vi "Automated Kitty Litter Box VI.vi"() -> ()   [LabVIEW 2021]
uses:
  <vilib>/LabVIEW Hacker/LINX/Private/Device/Type Defs/Stimulus Pulse.ctl
  <vilib>/LabVIEW Hacker/LINX/Public/Peripherals/Digital/Digital Write 1 Chan.vi
  <vilib>/Quanser/Rapid Control Prototyping Toolkit/hardware/HIL Board/_TypeSpecific/HIL Read Analog (Scalar).vi
  <vilib>/LabVIEW Hacker/LINX/LVH-LINX.lvlib
  <vilib>/Quanser/Rapid Control Prototyping Toolkit/hardware/HIL Board/HIL Board.lvclass
  <vilib>/LabVIEW Hacker/LINX/Private/Device/Device.lvlib
panel:
  out "Waveform Chart":dbl(graph)
  out "Rev":dbl
  out "Count":i32
  in  "stop":bool
  out "Distance (inches)":u32 format="%.2f"
  in  "Serial Port":refnum<visa-resource-name>="N/A"
  out "Saved Value":dbl
  out "Force Sensor Output":dbl
  # "FORCE SENSOR"
  # "MAIN MOTOR HALL EFFECT SENSOR"
  # "ULTRASONIC SENSOR"
  # "ARDUINO INITIALIZATION"
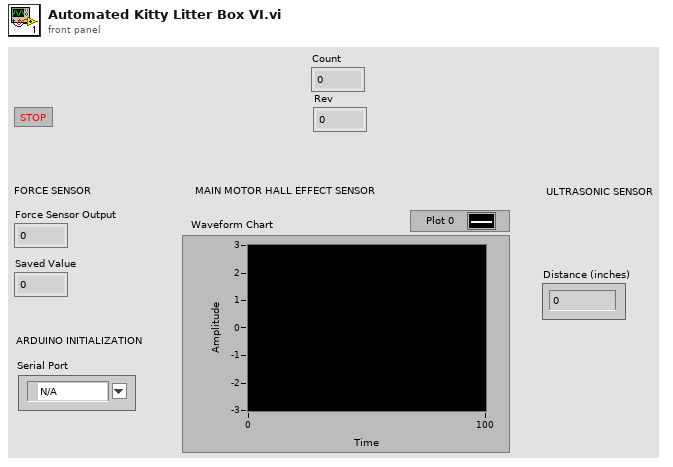
[diagram p1: front panel]
types:
  T1 = typedef "LVH-LINX.lvlib/LINX Ref.ctl" = cluster{"Platform":T2, "Interface":T3, "LINX Device Config":T4}
  T2 = typedef "LVH-LINX.lvlib/Platform.ctl" = enum16{"LINX", "myRIO"}
  T3 = typedef "LVH-LINX.lvlib/Interface.ctl" = enum16{"Serial", "TCP"}
  T4 = typedef "LVH-LINX.lvlib/Device.lvlib/LINX Device Config.ctl" = cluster{"Interface":T3, "COM Port":refnum<visa-resource-name>, "TCP Configuration":T5, "Device Family":T6, "Device ID":u8, "Device Name":string, "TCP Ref":refnum<k5>}
  T5 = typedef "LVH-LINX.lvlib/Device.lvlib/TCP Config.ctl" = cluster{"IP Address":string, "Port":u16}
  T6 = typedef "LVH-LINX.lvlib/Device Family.ctl" = enum8{"National Instruments", "Digilent", "Arduino"}
  T7 = typedef "LVH-LINX.lvlib/Device.lvlib/Stimulus Pulse.ctl" = enum16{"None", "Active Low", "Active High"}
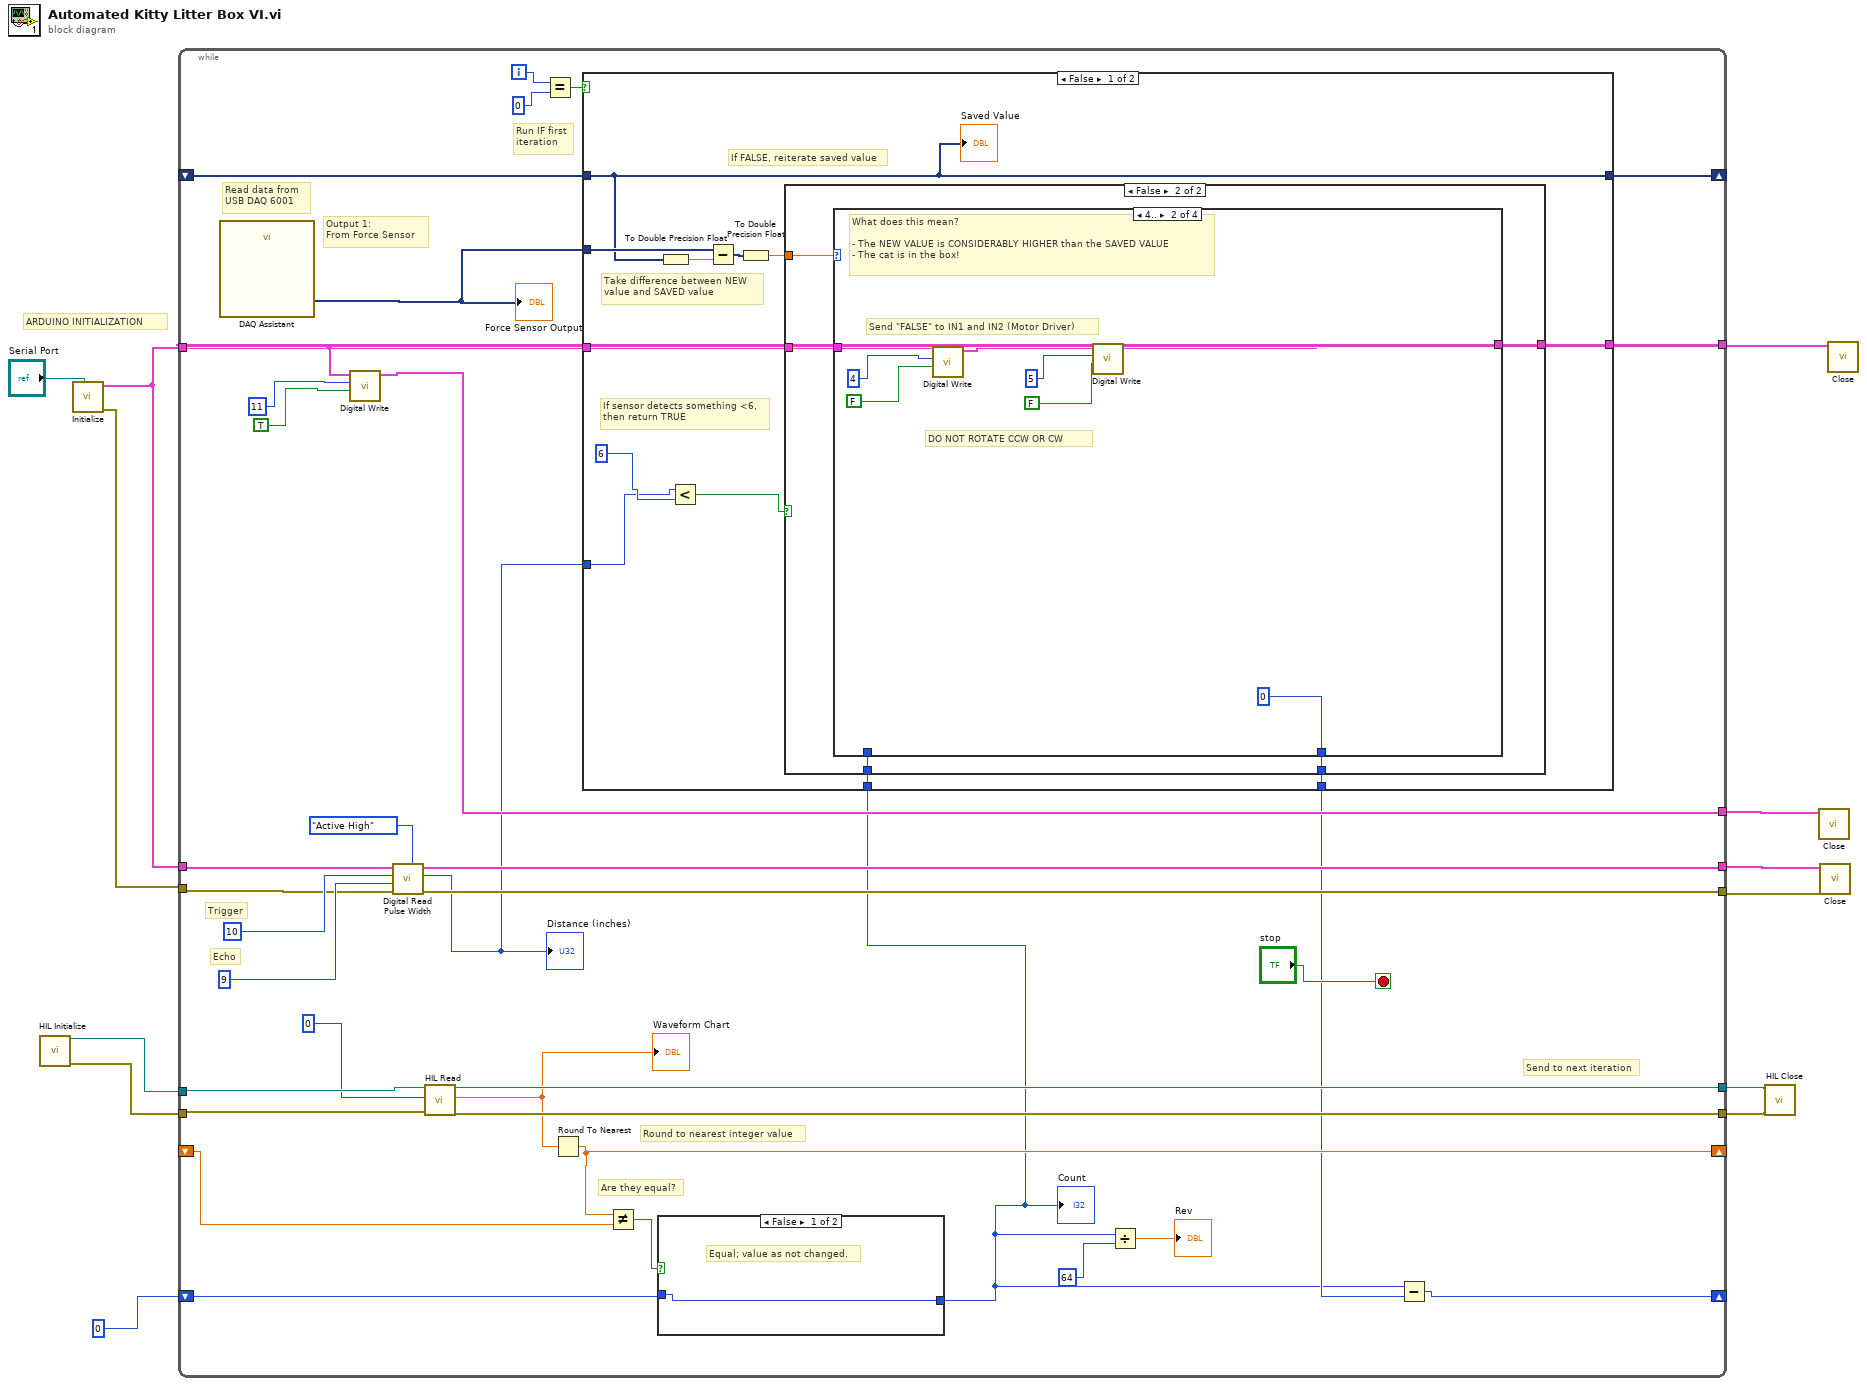
[diagram p0: block diagram]
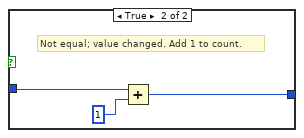
[diagram p2: hidden frame]
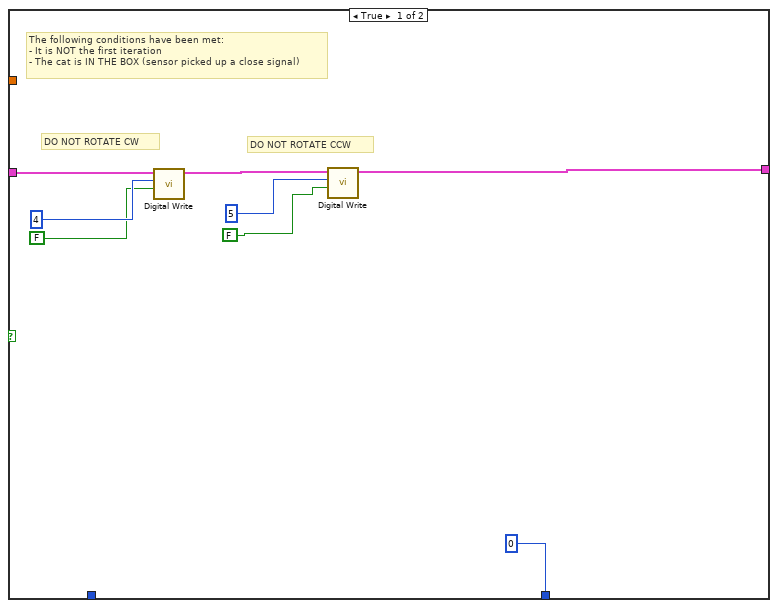
[diagram p3: hidden frame]
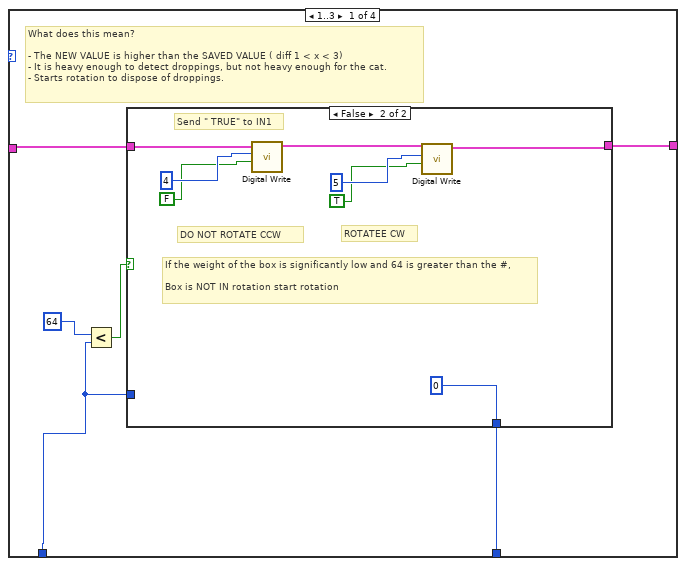
[diagram p4: hidden frame]
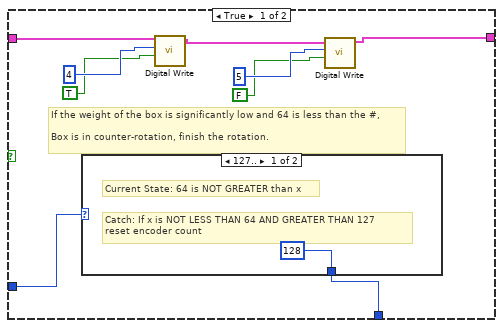
[diagram p5: hidden frame]
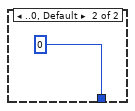
[diagram p6: hidden frame]
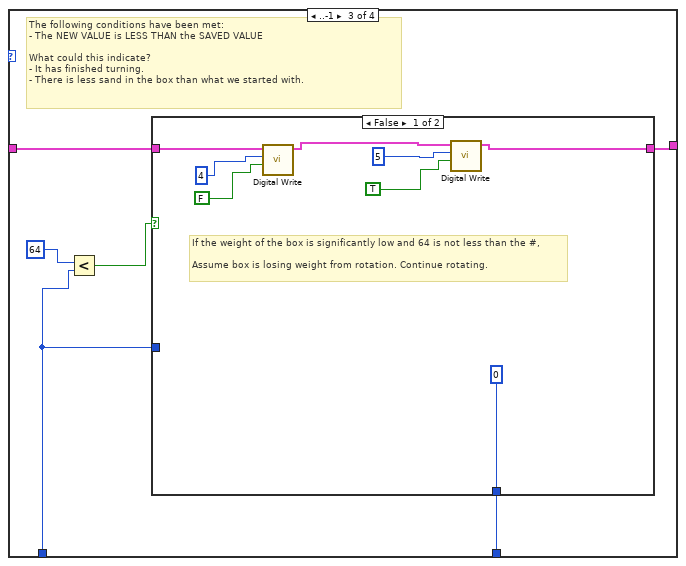
[diagram p7: hidden frame]
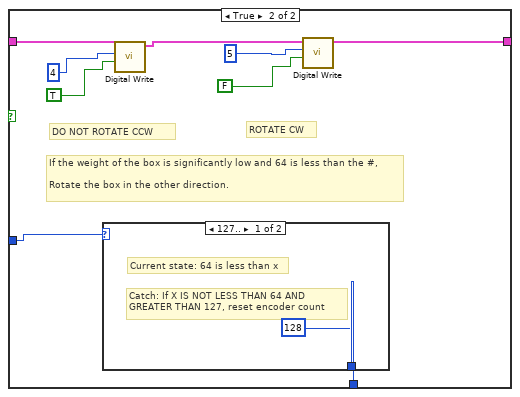
[diagram p8: hidden frame]
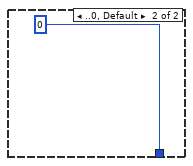
[diagram p9: hidden frame]
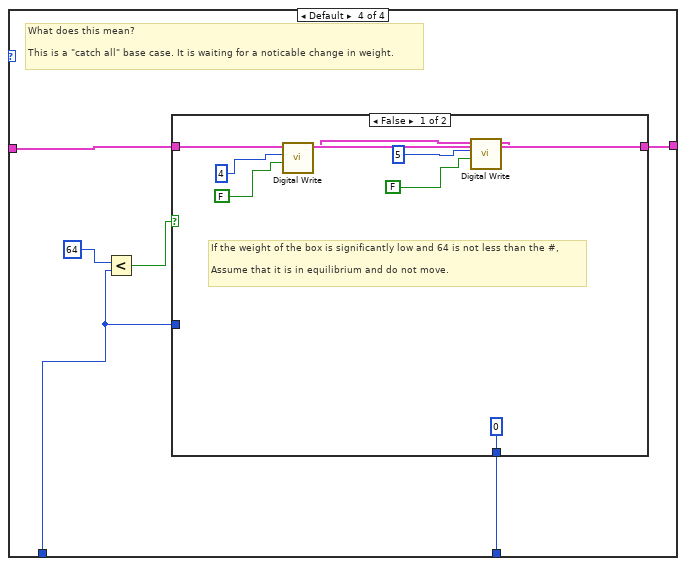
[diagram p10: hidden frame]
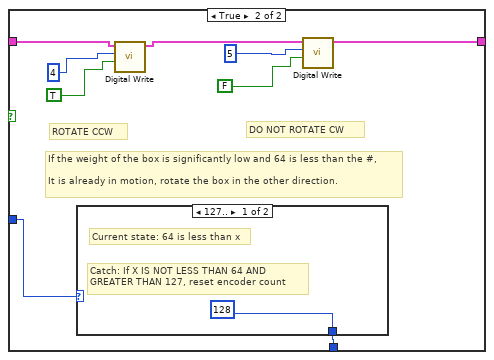
[diagram p11: hidden frame]
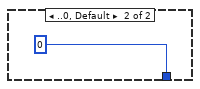
[diagram p12: hidden frame]
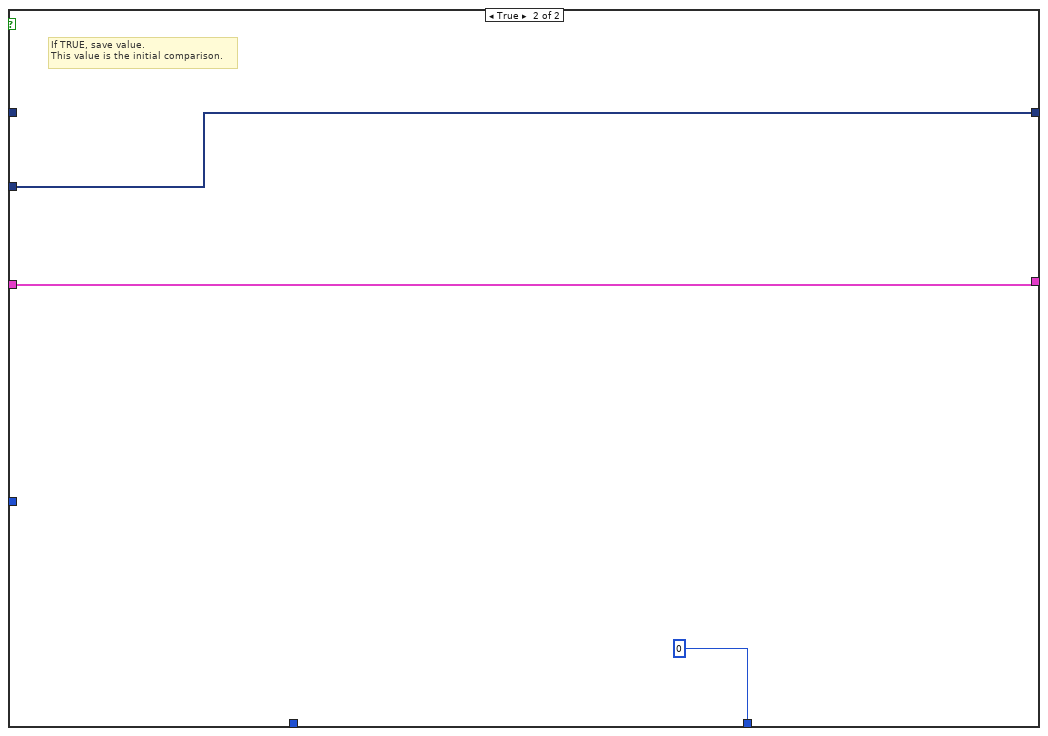
[diagram p13: hidden frame]
diagram:
  # "ARDUINO INITIALIZATION"
  n1 = call "HIL Initialize"() -> ("board out"=w5:refnum<class "HIL Board.lvclass">, "error out"=w4:errorcluster)  [unwired: 14 in]
  n2 = call <vilib>:"Initialize.vi"("Serial Port"="Serial Port") -> ("Error Out"=w8:errorcluster, "LINX Ref"=w10:T1)  [unwired: 8 in, 1 out]
  n3 = while {
    shift-right: [w44] -> _
    shift-left: _ -> [w43]
    tunnel: w10 -> [w27]
    tunnel: [w26] -> w7
    shift-right: [w15] -> _
    shift-left: 0 -> [w41]
    tunnel: w10 -> [w35]
    tunnel: [w34] -> w9
    tunnel: w8 -> [w23]
    tunnel: [w33] -> w6
    tunnel: w5 -> [w32]
    tunnel: w4 -> [w30]
    tunnel: [w29] -> w2
    tunnel: [w28] -> w3
    tunnel: [w22] -> w1
    shift-right: [w18] -> _
    shift-left: _ -> [w17]
    i -> [w47]
    stop <- "stop" stop-if-true
    # "Are they equal?"
    # "Send to next iteration"
    # "Round to nearest integer value"
    # "Trigger"
    # "Echo"
    # "Run IF first\niteration"
    # "Output 1:\nFrom Force Sensor"
    # "Read data from \nUSB DAQ 6001"
    n4 = call "DAQ Assistant"() -> ("data"=w38:dynamicdata)  [unwired: 17 in, 2 out]
    "Force Sensor Output" <- w38
    n5 = call-poly <vilib>:"Digital Write.vi"("Output Value"=TRUE, "DO Channel"=u8 11, "LINX Resource"=w35) -> ("LINX Resource"=w34:T1)  [unwired: 7 in, 1 out]
    n6 = call <vilib>:"Digital Read Pulse Width.vi"("Stimulus Pulse (Active High)"=Stimulus_Pulse."Active High", "Error In"=w23, "DO Channel"=9, "DI Channel"=10, "LINX Resource"=w27) -> ("Error Out"=w22:errorcluster, "Pulse Width (uS)"=w20:u32, "LINX Resource"=w26:T1)  [unwired: 4 in]
    "Distance (inches)" <- w20
    n7 = call-poly <vilib>:"HIL Read.vi"("board in"=w32, "channel"=0, "error in (no error)"=w30) -> ("board out"=w28:refnum<class "HIL Board.lvclass">, "voltage"=w19:dbl, "error out"=w29:errorcluster)  [unwired: 14 in]
    "Waveform Chart" <- w19
    n8 = Equal?(x=w47, y=0) -> (x = y?=w45:bool)
    n9 = Round To Nearest(number=w19) -> (nearest integer value=w18:dbl)
    n10 = Not Equal?(x=w18, y=w17) -> (x != y?=w16:bool)
    n11 = case shown="False" w16 {
      tunnel: [w48 w50] -> w13
      tunnel: w41 -> [w48 w49]
      frame False {
        # "Equal; value as not changed."
      }
      frame True {
        # "Not equal; value changed. Add 1 to count."
        n12 = Add(x=w49, y=1) -> (x+y=w50:i32)
      }
    }
    "Count" <- w13
    n13 = case shown="False" w45 {
      tunnel: w38 -> [w63 w161]
      tunnel: [w61 w161] -> w44
      tunnel: w43 -> [w61 _]
      tunnel: w35 -> [w58 w160]
      tunnel: w20 -> [w55 _]
      tunnel: [w54 w160] -> w33
      tunnel: w13 -> [w53 _]
      tunnel: [w52 0] -> w14
      frame False {
        # "If sensor detects something <6,\nthen return TRUE"
        # "Take difference between NEW\nvalue and SAVED value"
        # "If FALSE, reiterate saved value"
        n14 = To Double Precision Float(number=w61) -> (double precision float=w62:dbl)
        n15 = Less?(x=w55, y=6) -> (x < y?=w57:bool)
        n16 = Subtract(x=w63, y=w62) -> (x-y=w60:dynamicdata)
        n17 = To Double Precision Float(number=w60) -> (double precision float=w59:dbl)
        n18 = case shown="False" w57 {
          tunnel: w59 -> [_ w76]
          tunnel: w58 -> [w68 w75]
          tunnel: [w66 w74] -> w54
          tunnel: w53 -> [_ w73]
          tunnel: [0 w72] -> w52
          frame True {
            # "The following conditions have been met:\n- It is NOT the first iteration\n- The cat is IN THE BOX (sensor picked up a close signal)"
            # "DO NOT ROTATE CCW"
            # "DO NOT ROTATE CW"
            n19 = call-poly <vilib>:"Digital Write.vi"("Output Value"=FALSE, "DO Channel"=u8 4, "LINX Resource"=w68) -> ("LINX Resource"=w67:T1)  [unwired: 7 in, 1 out]
            n20 = call-poly <vilib>:"Digital Write.vi"("Output Value"=FALSE, "DO Channel"=u8 5, "LINX Resource"=w67) -> ("LINX Resource"=w66:T1)  [unwired: 7 in, 1 out]
          }
          frame False {
            n21 = case shown="4.." w76 {
              tunnel: w75 -> [w82 w108 w115 w137]
              tunnel: [w81 w109 w114 w137] -> w74
              tunnel: w73 -> [w77 _ w110 w135]
              tunnel: [w78 0 w111 w136] -> w72
              frame 1..3 {
                # "What does this mean?\n\n- The NEW VALUE is higher than the SAVED VALUE ( diff 1 < x < 3)\n- It is heavy enough to detect droppings, but not heavy enough for the cat.\n- Starts rotation to dispose of droppings."
                n22 = Less?(x=64, y=w77) -> (x < y?=w79:bool)
                n23 = case shown="False" w79 {
                  tunnel: w82 -> [w87 w101]
                  tunnel: [w85 w95] -> w81
                  tunnel: [w84 0] -> w78
                  tunnel: w77 -> [w83 _]
                  frame True {
                    # "If the weight of the box is significantly low and 64 is less than the #,\n\nBox is in counter-rotation, finish the rotation."
                    n24 = case shown="127.." w83 {
                      tunnel: [128 0] -> w84
                      frame 127.. {
                        # "Current State: 64 is NOT GREATER than x"
                        # "Catch: If x is NOT LESS THAN 64 AND GREATER THAN 127\nreset encoder count"
                      }
                      frame ..0, Default {
                      }
                    }
                    n25 = call-poly <vilib>:"Digital Write.vi"("Output Value"=TRUE, "DO Channel"=u8 4, "LINX Resource"=w87) -> ("LINX Resource"=w86:T1)  [unwired: 7 in, 1 out]
                    n26 = call-poly <vilib>:"Digital Write.vi"("Output Value"=FALSE, "DO Channel"=u8 5, "LINX Resource"=w86) -> ("LINX Resource"=w85:T1)  [unwired: 7 in, 1 out]
                  }
                  frame False {
                    # "If the weight of the box is significantly low and 64 is greater than the #,\n\nBox is NOT IN rotation start rotation"
                    # "ROTATEE CW"
                    # "DO NOT ROTATE CCW"
                    # "Send \" TRUE\" to IN1"
                    n27 = call-poly <vilib>:"Digital Write.vi"("Output Value"=FALSE, "DO Channel"=u8 4, "LINX Resource"=w101) -> ("LINX Resource"=w96:T1)  [unwired: 7 in, 1 out]
                    n28 = call-poly <vilib>:"Digital Write.vi"("Output Value"=TRUE, "DO Channel"=u8 5, "LINX Resource"=w96) -> ("LINX Resource"=w95:T1)  [unwired: 7 in, 1 out]
                  }
                }
              }
              frame 4.. {
                # "DO NOT ROTATE CCW OR CW"
                # "Send \"FALSE\" to IN1 and IN2 (Motor Driver)"
                # "What does this mean?\n\n- The NEW VALUE is CONSIDERABLY HIGHER than the SAVED VALUE\n- The cat is in the box!"
                n29 = call-poly <vilib>:"Digital Write.vi"("Output Value"=FALSE, "DO Channel"=u8 4, "LINX Resource"=w108) -> ("LINX Resource"=w107:T1)  [unwired: 7 in, 1 out]
                n30 = call-poly <vilib>:"Digital Write.vi"("Output Value"=FALSE, "DO Channel"=5, "LINX Resource"=w107) -> ("LINX Resource"=w109:T1)  [unwired: 7 in, 1 out]
              }
              frame ..-1 {
                # "The following conditions have been met:\n- The NEW VALUE is LESS THAN the SAVED VALUE\n\nWhat could this indicate?\n- It has finished turning.\n- There is less sand in the box than what we started with."
                n31 = Less?(x=64, y=w110) -> (x < y?=w112:bool)
                n32 = case shown="False" w112 {
                  tunnel: w115 -> [w119 w132]
                  tunnel: [w117 w130] -> w114
                  tunnel: [0 w124] -> w111
                  tunnel: w110 -> [_ w125]
                  frame False {
                    # "If the weight of the box is significantly low and 64 is not less than the #,\n\nAssume box is losing weight from rotation. Continue rotating."
                    n33 = call-poly <vilib>:"Digital Write.vi"("Output Value"=FALSE, "DO Channel"=u8 4, "LINX Resource"=w119) -> ("LINX Resource"=w118:T1)  [unwired: 7 in, 1 out]
                    n34 = call-poly <vilib>:"Digital Write.vi"("Output Value"=TRUE, "DO Channel"=5, "LINX Resource"=w118) -> ("LINX Resource"=w117:T1)  [unwired: 7 in, 1 out]
                  }
                  frame True {
                    # "If the weight of the box is significantly low and 64 is less than the #,\n\nRotate the box in the other direction."
                    # "ROTATE CW"
                    # "DO NOT ROTATE CCW"
                    n35 = case shown="127.." w125 {
                      tunnel: [128 0] -> w124
                      frame 127.. {
                        # "Current state: 64 is less than x"
                        # "Catch: If X IS NOT LESS THAN 64 AND \nGREATER THAN 127, reset encoder count"
                      }
                      frame ..0, Default {
                      }
                    }
                    n36 = call-poly <vilib>:"Digital Write.vi"("Output Value"=TRUE, "DO Channel"=u8 4, "LINX Resource"=w132) -> ("LINX Resource"=w131:T1)  [unwired: 7 in, 1 out]
                    n37 = call-poly <vilib>:"Digital Write.vi"("Output Value"=FALSE, "DO Channel"=5, "LINX Resource"=w131) -> ("LINX Resource"=w130:T1)  [unwired: 7 in, 1 out]
                  }
                }
              }
              frame Default {
                # "What does this mean?\n\nThis is a \"catch all\" base case. It is waiting for a noticable change in weight."
                n38 = Less?(x=64, y=w135) -> (x < y?=w138:bool)
                n39 = case shown="False" w138 {
                  tunnel: [w142 w155] -> _
                  tunnel: w137 -> [w141 w150]
                  tunnel: [0 w148] -> w136
                  tunnel: w135 -> [_ w149]
                  frame False {
                    # "If the weight of the box is significantly low and 64 is not less than the #,\n\nAssume that it is in equilibrium and do not move."
                    n40 = call-poly <vilib>:"Digital Write.vi"("Output Value"=FALSE, "DO Channel"=u8 4, "LINX Resource"=w141) -> ("LINX Resource"=w143:T1)  [unwired: 7 in, 1 out]
                    n41 = call-poly <vilib>:"Digital Write.vi"("Output Value"=FALSE, "DO Channel"=5, "LINX Resource"=w143) -> ("LINX Resource"=w142:T1)  [unwired: 7 in, 1 out]
                  }
                  frame True {
                    # "If the weight of the box is significantly low and 64 is less than the #,\n\nIt is already in motion, rotate the box in the other direction."
                    # "DO NOT ROTATE CW"
                    # "ROTATE CCW"
                    n42 = case shown="127.." w149 {
                      tunnel: [128 0] -> w148
                      frame 127.. {
                        # "Current state: 64 is less than x"
                        # "Catch: If X IS NOT LESS THAN 64 AND \nGREATER THAN 127, reset encoder count"
                      }
                      frame ..0, Default {
                      }
                    }
                    n43 = call-poly <vilib>:"Digital Write.vi"("Output Value"=TRUE, "DO Channel"=u8 4, "LINX Resource"=w150) -> ("LINX Resource"=w156:T1)  [unwired: 7 in, 1 out]
                    n44 = call-poly <vilib>:"Digital Write.vi"("Output Value"=FALSE, "DO Channel"=5, "LINX Resource"=w156) -> ("LINX Resource"=w155:T1)  [unwired: 7 in, 1 out]
                  }
                }
              }
            }
          }
        }
        "Saved Value" <- w61
      }
      frame True {
        # "If TRUE, save value.\nThis value is the initial comparison."
      }
    }
    n45 = Divide(x=w13, y=64) -> (x/y=→"Rev":dbl)
    n46 = Subtract(x=w13, y=w14) -> (x-y=w15:i32)
  }
  n47 = call <vilib>:"HIL Close.vi"("error in (no error)"=w2, "board in"=w3) -> ()  [unwired: 9 in, 1 out]
  n48 = call <vilib>:"Close.vi"("LINX Resource"=w9) -> ()  [unwired: 9 in, 2 out]
  n49 = call <vilib>:"Close.vi"("Error In"=w1, "LINX Resource"=w7) -> ()  [unwired: 8 in, 2 out]
  n50 = call <vilib>:"Close.vi"("LINX Resource"=w6) -> ()  [unwired: 9 in, 2 out]
